vi "Test Helper Loop Restart.vi"(8 "error in (no error)":errorcluster, 11 "Helper Loop Test In":refnum<class "Helper Loop Test.lvclass">) -> (0 "error out":errorcluster, 3 "Helper Loop Test Out":refnum<class "Helper Loop Test.lvclass">)   [LabVIEW 2020, in "Helper Loop Test.lvclass"]
uses:
  Helper Loop Test.lvclass
  C:/Program Files (x86)/National Instruments/LabVIEW 2020/vi.lib/Astemes/LUnit/Test Case.lvclass
  source/Framework Test Suite/Mock Process/Mock Process.lvclass
  C:/Git/astemes-triarc-framework/source/Framework/Process/Process.lvclass
  source/Framework/Process/Process.lvclass/Process.ctl
  <vilib>/Astemes/LUnit/Test Case.lvclass/Test Case.ctl
  <vilib>/Astemes/LUnit/LUnit Assertion Result.lvclass/LUnit Assertion Result.ctl
  <vilib>/Astemes/LUnit/LUnit Test Case Result.lvclass/LUnit Test Case Result.ctl
  <vilib>/Astemes/LUnit/LUnit Method Result.lvclass/LUnit Method Result.ctl
  5c824806-a2a3-41ed-ad4d-6f7d99db2d3e.vi
  f58b967f-3bde-4b6b-a42a-cab2bdf802bc.vi
  source/Framework/Process/Public/Lifecycle/Get Lifecycle State.vi
  source/Framework/Broadcast Event Helpers/Execution timer.vi
  <vilib>/Astemes/LUnit/Palette/Pass.vi
  <vilib>/Astemes/LUnit/Palette/Fail.vi
  <vilib>/Astemes/LUnit/Compare Variants.vi
  <vilib>/Astemes/LUnit/Describe Comparison.vi
  <vilib>/Astemes/LUnit/Set Assertion Type.vi
  source/Framework/Process/Private/SubVIs/Wait for finish.vi
  source/Framework/Process/Protected/Messaging/Enqueue Message.vi
  source/Framework/Process/Private/SubVIs/Set Lifecycle State.vi
  <vilib>/Utility/error.llb/Clear Errors.vi
  <vilib>/Astemes/LUnit/Add test result.vi
  <vilib>/Astemes/LUnit/LUnit Write Passed.vi
  <vilib>/Astemes/LUnit/LUnit Write Message.vi
  <vilib>/Astemes/LUnit/LUnit Write Description.vi
  <vilib>/Astemes/LUnit/Variant to string.vi
  <vilib>/Astemes/LUnit/LUnit Write Assertion Type.vi
  source/Framework/Process/Private/SubVIs/Handle Debug Data.vi
  <vilib>/Astemes/LUnit/LUnit Record Assertion Result.vi
  source/Framework/Logging/Log Debug.vi
  <vilib>/AdvancedString/1D String Array to Delimited String.vi
  <vilib>/Utility/High Resolution Relative Seconds.vi
  <vilib>/Astemes/LUnit/LUnit Aggregate Assertion Results.vi
  <vilib>/Astemes/LUnit/Assertion Result/LUnit Read Status.vi
  <vilib>/Astemes/LUnit/LUnit Read Message.vi
  <vilib>/Astemes/LUnit/LUnit Read Description.vi
  <vilib>/Astemes/LUnit/Method Result/LUnit Merge Status.vi
  <vilib>/Astemes/LUnit/LUnit Concatenate result strings.vi
  <vilib>/Utility/error.llb/Error Cluster From Error Code.vi
  source/Framework/Broadcast Event Helpers/Dequeue Broadcast Message.vi
  <vilib>/Utility/Data Type/Get Type Information.vi
  <vilib>/Utility/LVClass/Get LV Class Name.vi
  source/Framework/Process/Public/Read Name.vi
  <vilib>/Astemes/LUnit/LUnit Assertion Result.lvclass
  source/Framework/Process/Process.lvclass
  source/Framework/Broadcast Event Helpers/Broadcast Event Helpers.lvlib
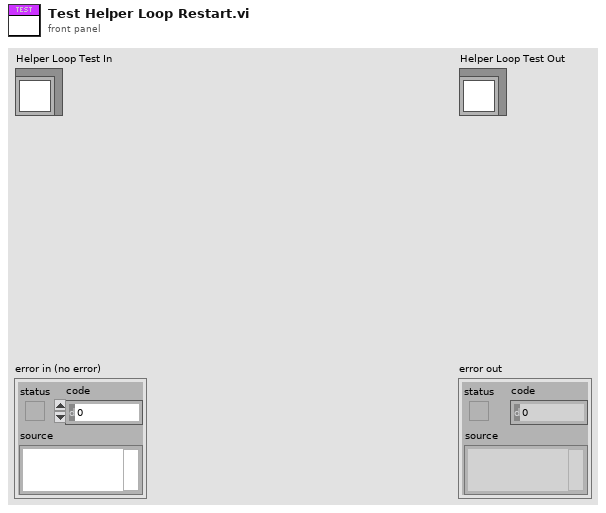
[diagram p1: front panel]
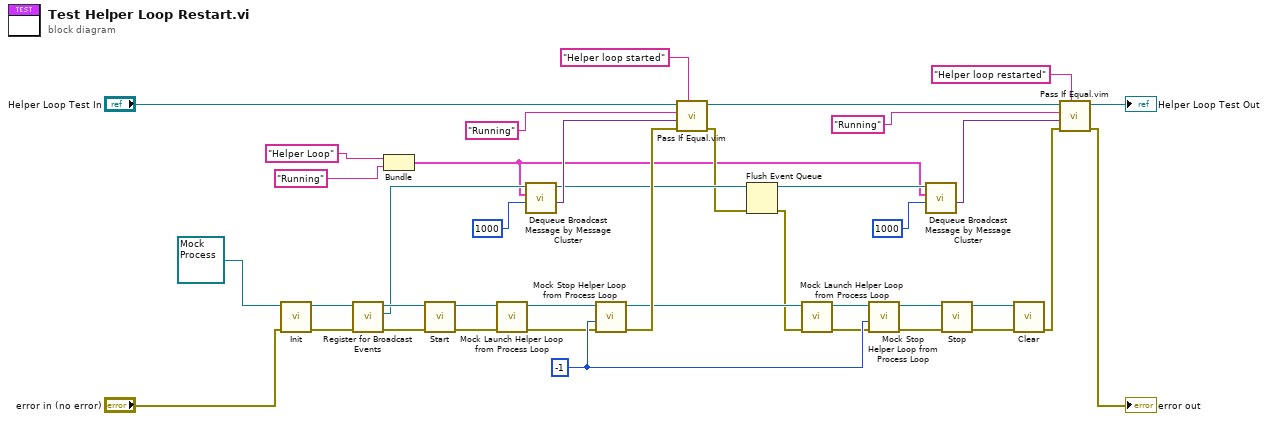
[diagram p0: block diagram]
diagram:
  w23 = -1 ("timeout in ms (-1)")
  n1 = call-dynamic "Init.vi"("error in (no error)"="error in (no error)", "Mock Process In"=refnum<class "Mock Process.lvclass"> refnum) -> ("error out"=w40:errorcluster, "Mock Process Out"=w20:refnum<class "Mock Process.lvclass">)  [unwired: 8 in]
  n2 = call "Register for Broadcast Events.vi"("error in (no error)"=w40, "Process In"=w20) -> ("error out"=w21:errorcluster, "Event Registration Refnum Out"=w13:refnum<event-registration>, "Process Out"=w19:refnum<class "Mock Process.lvclass">)  [unwired: 7 in]
  n3 = Bundle("y"="Helper Loop", "Description"="Running") -> (w1:cluster{"y":string, "Description":string})  [unwired: 1 in]
  n4 = call "Start.vi"("error in (no error)"=w21, "Process In"=w19) -> ("error out"=w38:errorcluster, "Process Out"=w39:refnum<class "Mock Process.lvclass">)  [unwired: 7 in, 1 out]
  n5 = call "Mock Launch Helper Loop from Process Loop.vi"("error in (no error)"=w38, "Mock Process in"=w39) -> ("error out"=w16:errorcluster, "Mock Process out"=w17:refnum<class "Mock Process.lvclass">)  [unwired: 8 in]
  n6 = call "Dequeue Broadcast Message by Message Cluster.vi"("Timeout (-1)"=1000, "Message"=w1, "Event Registration Refnum"=w13) -> ("Message Data"=w12:variant, "Event Registration Refnum Out"=w8:refnum<event-registration>)  [unwired: 4 in, 3 out]
  n7 = call "Mock Stop Helper Loop from Process Loop.vi"("error in (no error)"=w16, "timeout in ms (-1)"=w23, "Mock Process in"=w17) -> ("error out"=w27:errorcluster, "Mock Process out"=w26:refnum<class "Mock Process.lvclass">)  [unwired: 6 in, 1 out]
  n8 = call "Pass If Equal.vim"("Description"="Helper loop started", "error in (no error)"=w27, "Actual"=w12, "Expected"="Running", "LUnit Test Case In"="Helper Loop Test In") -> ("error out"=w7:errorcluster, "LUnit Test Case Out"=w29:refnum<class "Helper Loop Test.lvclass">)  [unwired: 5 in]
  n9 = Flush Event Queue(0:w8, 3:w7) -> (8:w9:refnum<event-registration>, 11:w6:errorcluster)  [unwired: 4 in, 1 out]
  n10 = call "Mock Launch Helper Loop from Process Loop.vi"("error in (no error)"=w6, "Mock Process in"=w26) -> ("error out"=w14:errorcluster, "Mock Process out"=w15:refnum<class "Mock Process.lvclass">)  [unwired: 8 in]
  n11 = call "Mock Stop Helper Loop from Process Loop.vi"("error in (no error)"=w14, "timeout in ms (-1)"=w23, "Mock Process in"=w15) -> ("error out"=w24:errorcluster, "Mock Process out"=w25:refnum<class "Mock Process.lvclass">)  [unwired: 6 in, 1 out]
  n12 = call "Dequeue Broadcast Message by Message Cluster.vi"("Timeout (-1)"=1000, "Message"=w1, "Event Registration Refnum"=w9) -> ("Message Data"=w5:variant)  [unwired: 4 in, 4 out]
  n13 = call "Stop.vi"("error in (no error)"=w24, "Process In"=w25) -> ("error out"=w37:errorcluster, "Process Out"=w22:refnum<class "Mock Process.lvclass">)  [unwired: 7 in, 1 out]
  n14 = call-dynamic "Clear.vi"("error in (no error)"=w37, "Mock Process In"=w22) -> ("error out"=w36:errorcluster)  [unwired: 9 in]
  n15 = call "Pass If Equal.vim"("Description"="Helper loop restarted", "error in (no error)"=w36, "Actual"=w5, "Expected"="Running", "LUnit Test Case In"=w29) -> ("error out"=→"error out":errorcluster, "LUnit Test Case Out"=→"Helper Loop Test Out":refnum<class "Helper Loop Test.lvclass">)  [unwired: 5 in]
